vi "单步启动对话框.vi"() -> (3 "单步启动步骤输出":u16)   [LabVIEW 2016, in "PLC.lvlib"]
uses:
  PLC.lvlib
panel:
  in  "取消":bool
  in  "确定":bool
  in  "单步启动步骤":u16(ring) items=["待机", "初始化", "水样润洗", "一级水样池进样", "沉淀", "二级水样池进样", "配水", "反冲洗", "采样池储水", "结束"]
  # "请选择要启动的步骤"
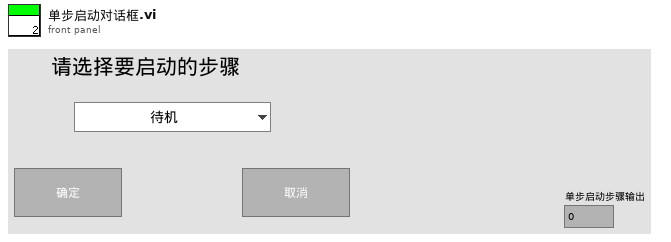
[diagram p1: front panel]
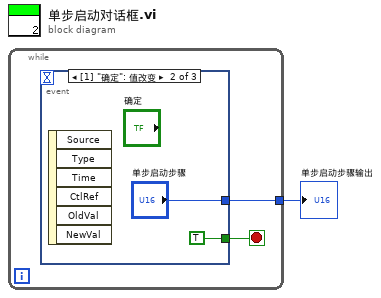
[diagram p0: block diagram]
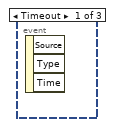
[diagram p2: hidden frame]
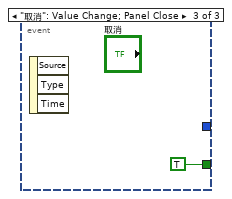
[diagram p3: hidden frame]
diagram:
  n1 = while {
    tunnel: [w2] -> w1
    stop <- w3 stop-if-true
    n2 = event shown="[1] \"确定\": 值改变" {
      selector: _ -> [_ _ _]
      dyn-events: _ -> [_ _ _]
      timeout: _ -> [_ _ _]
      tunnel: [_ TRUE TRUE] -> w3
      tunnel: [_ "单步启动步骤" _] -> w2
      event Timeout {
        n3 = event-data() -> ()  [unwired: 1 in, 3 out]
      }
      event "确定": Value Change {
        n4 = event-data() -> ()  [unwired: 1 in, 6 out]
      }
      event "取消": Value Change; Panel Close {
        n5 = event-data() -> ()  [unwired: 1 in, 3 out]
      }
    }
  }
  "单步启动步骤输出" <- w1
